vi "Calculate N_total and Updates.vi"(2 "Configuration.DAQ.Sampling.Sampling":T1={"Fs"=204789.0, "#s"=15753} {"Fs" format="%#_13g"}, 3 "Sweep Time (s)":dbl) -> (0 "Updates":i32, 1 "N_Total":i32)   [LabVIEW 2019, in "Instrument.Lockin.lvlib" / "Instrument.DAQ.lvclass"]
uses:
  Instrument.DAQ.lvclass
  Typedefs/DAQ.Sampling.Sampling--Cluster.ctl
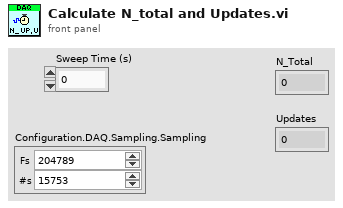
[diagram p1: front panel]
types:
  T1 = typedef "Instrument.Lockin.lvlib/Instrument.DAQ.lvclass/DAQ.Sampling.Sampling--Cluster.ctl" = cluster{"Fs":dbl, "#s":i32}
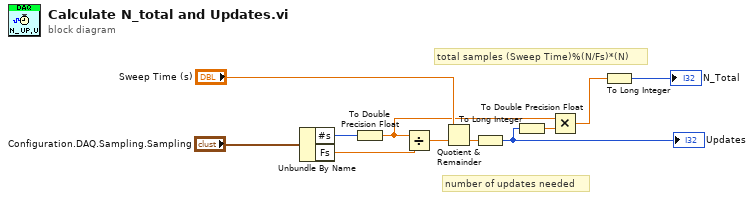
[diagram p0: block diagram]
diagram:
  # "number of updates needed"
  # "total samples (Sweep Time)%(N/Fs)*(N)"
  n1 = Unbundle By Name("Configuration.DAQ.Sampling.Sampling") -> ("#s"=w9:i32, "Fs"=w8:dbl)
  n2 = To Double Precision Float(number=w9) -> (double precision float=w3:dbl)
  n3 = Divide(x=w3, y=w8) -> (x/y=w6:dbl)
  n4 = Quotient & Remainder(x="Sweep Time (s)", y=w6) -> (floor(x/y)=w7:dbl)  [unwired: 1 out]
  n5 = To Long Integer(number=w7) -> (32bit integer=w10:i32)
  "Updates" <- w10
  n6 = To Double Precision Float(number=w10) -> (double precision float=w1:dbl)
  n7 = Multiply(x=w3, y=w1) -> (x*y=w11:dbl)
  n8 = To Long Integer(number=w11) -> (32bit integer=→"N_Total":i32)
